vi "Untitled 1.vi"   [LabVIEW 2021]
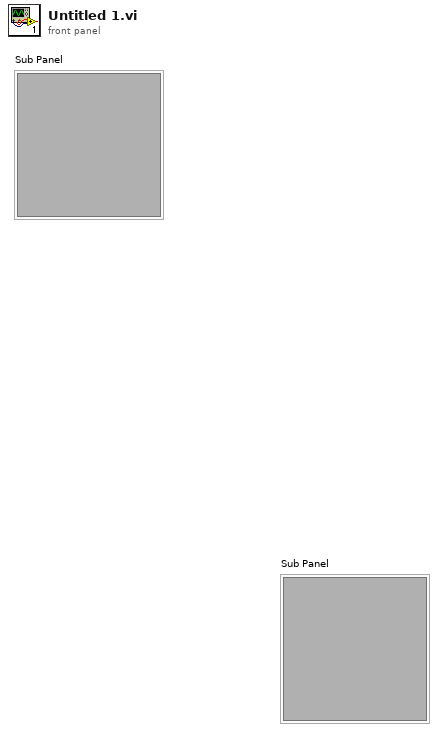
[diagram p1: front panel]
types:
  T1 = enum32{"Invalid", "Standard", "Closed", "Hidden", "Minimized", "Maximized"}
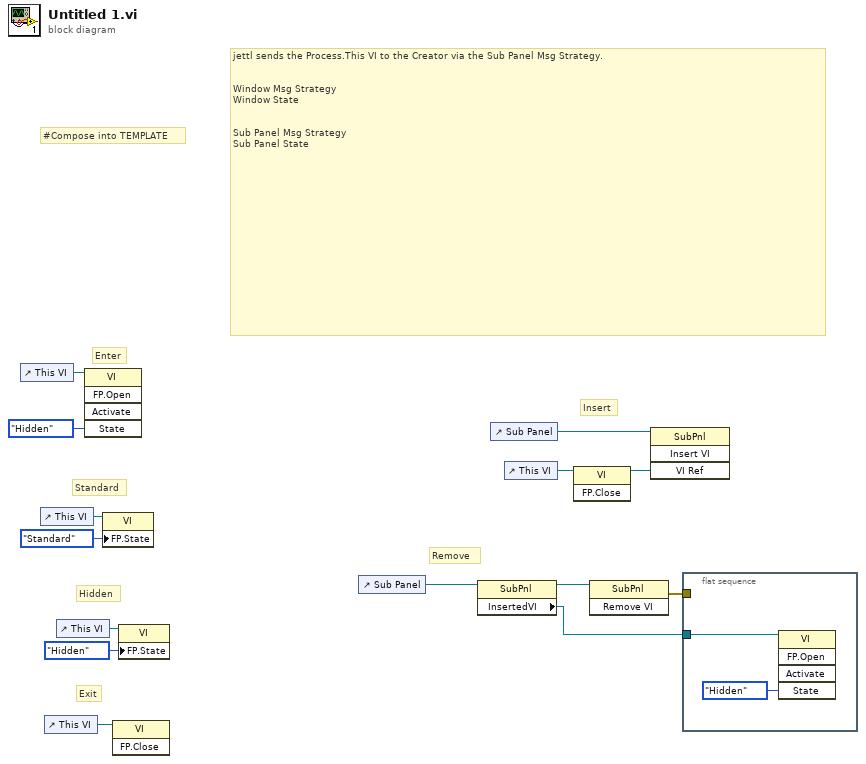
[diagram p0: block diagram]
diagram:
  # "Exit"
  # "Standard"
  # "Enter"
  # "Hidden"
  # "Remove"
  # "Insert"
  # "jettl sends the Process.This VI to the Creator via the Sub Panel Msg Strategy.\n\n\nWindow Msg Strategy\nWindow State\n\n\nSub Panel Msg Strategy\nSub Panel State"
  # "#Compose into TEMPLATE"
  n1 = control-ref of="This VI"() -> (w11:refnum<vi>)
  n2 = control-ref of="This VI"() -> (w9:refnum<vi>)
  n3 = control-ref of="This VI"() -> (w10:refnum<vi>)
  n4 = control-ref of="This VI"() -> (w6:refnum<vi>)
  n5 = invoke class="VI" method="FP.Open"(reference=w11, "State"=T1."Hidden") -> ()  [unwired: 3 in, 5 out]
  n6 = property class="VI"(reference=w9, "FP.State"=T1."Standard" ("Front Panel Window:State")) -> ()  [unwired: 1 in, 2 out]
  n7 = invoke class="VI" method="FP.Close"(reference=w10) -> ()  [unwired: 2 in, 3 out]
  n8 = property class="VI"(reference=w6, "FP.State"=T1."Hidden" ("Front Panel Window:State")) -> ()  [unwired: 1 in, 2 out]
  n9 = control-ref of="Sub Panel"() -> (w5:refnum<vi>)
  n10 = property class="SubPnl"(reference=w5) -> (reference out=w4:refnum<vi>, "InsertedVI"=w3:refnum<vi>)  [unwired: 1 in, 1 out]
  n11 = control-ref of="Sub Panel"() -> (w14:refnum<vi>)
  n12 = control-ref of="This VI"() -> (w13:refnum<vi>)
  n13 = invoke class="VI" method="FP.Close"(reference=w13) -> (reference out=w2:refnum<vi>)  [unwired: 2 in, 2 out]
  n14 = invoke class="SubPnl" method="Remove VI"(reference=w4) -> (error out=w1:errorcluster)  [unwired: 2 in, 2 out]
  n15 = invoke class="SubPnl" method="Insert VI"(reference=w14, "VI Ref"=w2) -> ()  [unwired: 2 in, 4 out]
  n16 = flat-sequence {
    tunnel: w3 -> [w15]
    tunnel: w1 -> [_]
    frame #0 {
      n17 = invoke class="VI" method="FP.Open"(reference=w15, "State"=T1."Hidden") -> ()  [unwired: 3 in, 5 out]
    }
  }
